vi "LVProjectShortcut_CreateNewWizard_IncludeItem.vi"(11 "Wizard":T1) -> (3 "Include me":bool)   [LabVIEW 2017]
uses:
  <resource>/Framework/Providers/API/ItemRef.ctl
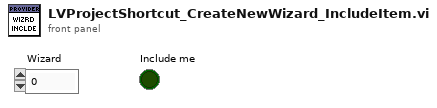
[diagram p1: front panel]
types:
  T1 = typedef "ItemRef.ctl" = u64
  T2 = typedef "mxLvNIIM.ctl" = cluster{"Item URL":string, "Item ID":string, "Item Index":i32, "Specific Type":string}
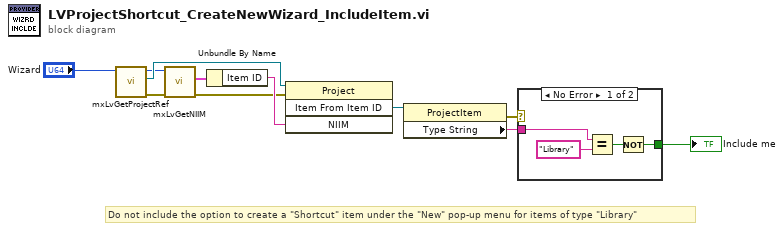
[diagram p0: block diagram]
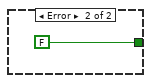
[diagram p2: hidden frame]
diagram:
  # "Do not include the option to create a \"Shortcut\" item under the \"New\" pop-up menu for items of type \"Library\""
  n1 = call <resource>:"mxLvGetProjectRef.vi"("Item"="Wizard") -> ("error out"=w5:errorcluster, "Project Refnum"=w8:refnum<vi>, "Item"=w2:T1)  [unwired: 8 in]
  n2 = call <resource>:"mxLvGetNIIM.vi"("error in"=w5, "Item"=w2) -> ("error out"=w4:errorcluster, "NIIM"=w11:T2)  [unwired: 7 in, 1 out]
  n3 = Unbundle By Name(w11) -> ("Item ID"=w10:string)
  n4 = invoke class="Project" method="Item From Item ID"(reference=w8, error in=w4, "NIIM"=w10) -> ("GetItemFromNIIM"=w9:refnum<vi>)  [unwired: 1 in, 3 out]
  n5 = property class="ProjectItem"(reference=w9) -> (error out=w7:errorcluster, "Type String"=w6:string)  [unwired: 1 in, 1 out]
  n6 = case shown="No Error" w7 {
    tunnel: w6 -> [w14 _]
    tunnel: [w12 FALSE] -> w1
    frame No Error {
      n7 = Equal?(x=w14, y="Library") -> (x = y?=w13:bool)
      n8 = Not(x=w13) -> (.not. x?=w12:bool)
    }
    frame Error {
    }
  }
  "Include me" <- w1
